vi "json Insert.vi"(8 "error in (no error)":errorcluster, 9 "anything":variant, 10 "path":string, 11 "JSON Document in":refnum<class "JSON Document.lvclass">) -> (0 "error out":errorcluster, 1 "replaced?":bool, 3 "JSON Document out":refnum<class "JSON Document.lvclass">)   [LabVIEW 2015, in "JSON Document.lvclass"]
uses:
  JSON Document.lvclass
  poly instances/json Insert I32 - string path.vi
  poly instances/json Insert I64 - string path.vi
  poly instances/json Insert U32 - string path.vi
  poly instances/json Insert U64 - string path.vi
  poly instances/json Insert Float - string path.vi
  poly instances/json Insert Double - string path.vi
  poly instances/json Insert Boolean - string path.vi
  poly instances/json Insert String - string path.vi
  poly instances/json Insert Path - string path.vi
  poly instances/json Insert json - string path.vi
  <vilib>/Utility/Data Type/NI_Data Type.lvlib
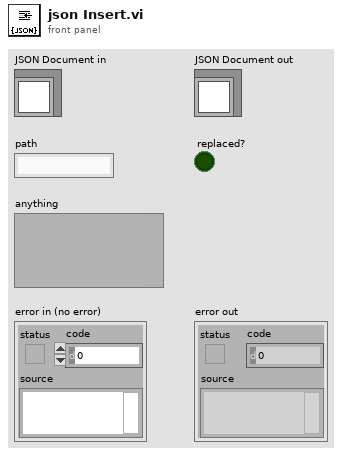
[diagram p1: front panel]
types:
  T1 = typedef "NI_Data Type.lvlib/Data Type.ctl" = enum8{"Invalid Type", "Void", "I8", "I16", "I32", "I64", "U8", "U16", "U32", "U64", "Single Float", "Double Float", "Extended Float", "Single Complex", "Double Complex", "Extended Complex", "Enum U8", "Enum U16", "Enum U32", "Enum U64", "Single Float With Unit", "Double Float With Unit", "Extended Float With Unit", "Single Complex with Unit", "Double Complex with Unit", "Extended Complex with Unit", "Boolean", "String", "Path", "Picture", "Tag", "Array", "Cluster", "Variant", "LV Variant", "Waveform", "Timestamp", "Digital Waveform", "Digital Data", "ExpressData", "Refnum", "External Data", "VI", "Poly VI", "LabVIEW Class Instance", "Fixed Point"}
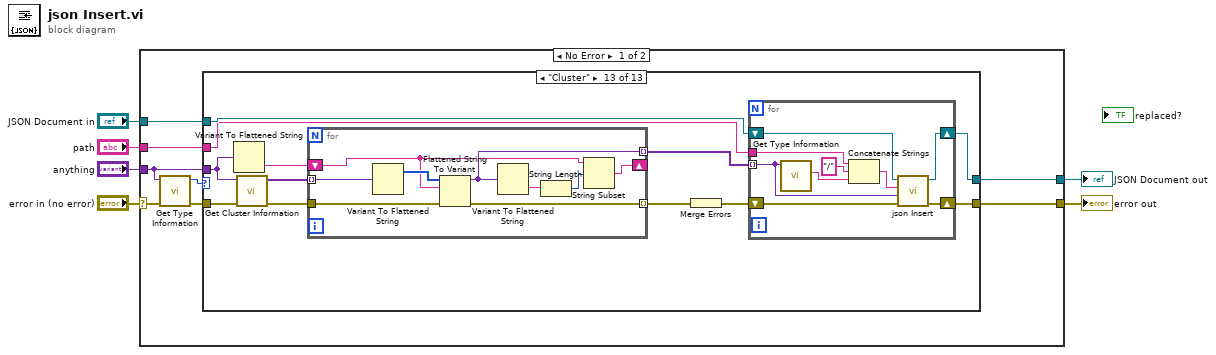
[diagram p0: block diagram]
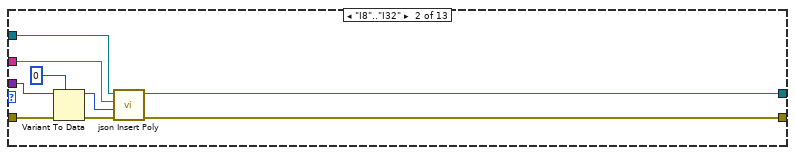
[diagram p3: hidden frame]
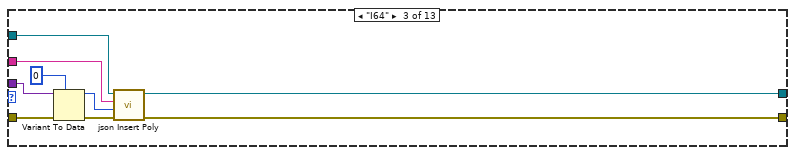
[diagram p4: hidden frame]
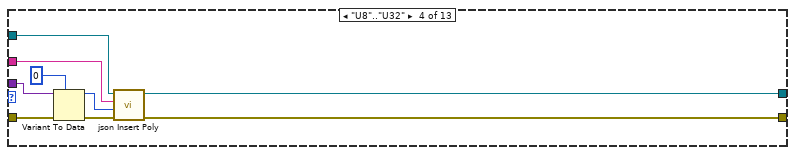
[diagram p5: hidden frame]
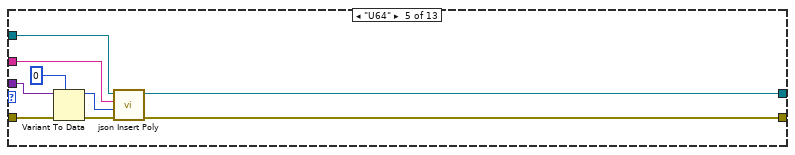
[diagram p6: hidden frame]
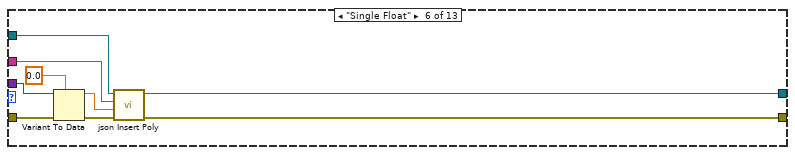
[diagram p7: hidden frame]
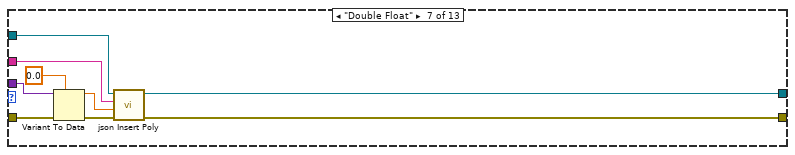
[diagram p8: hidden frame]
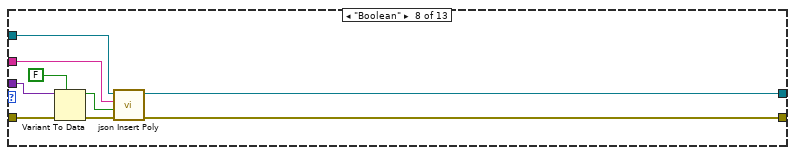
[diagram p9: hidden frame]
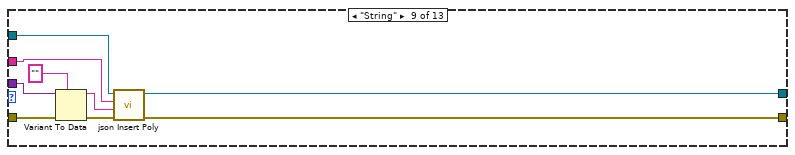
[diagram p10: hidden frame]
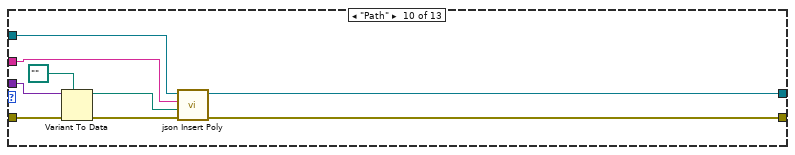
[diagram p11: hidden frame]
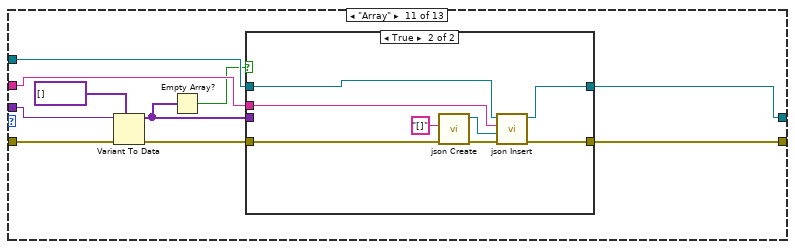
[diagram p12: hidden frame]
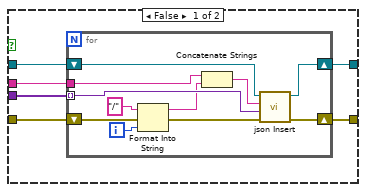
[diagram p13: hidden frame]
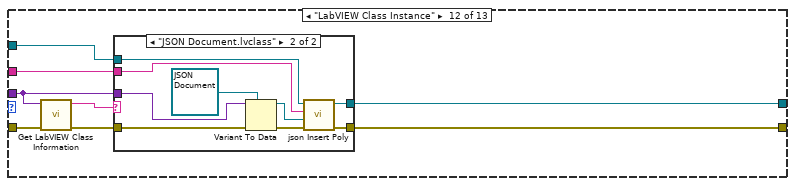
[diagram p14: hidden frame]
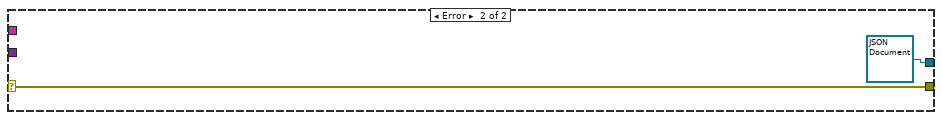
[diagram p16: hidden frame]
diagram:
  n1 = case shown="No Error" "error in (no error)" {
    selector: "error in (no error)" -> [w10 w182]
    tunnel: "anything" -> [w13 _]
    tunnel: [w11 refnum<class "JSON Document.lvclass"> refnum ("JSON Document out")] -> w4
    tunnel: [w9 w182] -> w3
    tunnel: "JSON Document in" -> [w8 _]
    tunnel: "path" -> [w7 _]
    frame No Error {
      n2 = call <vilib>:"Get Type Information.vi"("error in (no error)"=w10, "Variant"=w13) -> ("error out"=w12:errorcluster, "Type"=w14:T1)  [unwired: 5 in, 3 out]
      n3 = case shown="\"Cluster\"" w14 {
        tunnel: w13 -> [_ w24 w33 w42 w51 w60 w69 w78 w87 w96 w106 w138 w159]
        tunnel: w12 -> [w16 w23 w32 w41 w50 w59 w68 w77 w86 w95 w105 w140 w153]
        tunnel: w8 -> [w15 w21 w30 w39 w48 w57 w66 w75 w84 w93 w103 w136 w156]
        tunnel: [w15 w19 w28 w37 w46 w55 w64 w73 w82 w91 w102 w133 w155] -> w11
        tunnel: [w16 w18 w27 w36 w45 w54 w63 w72 w81 w90 w101 w134 w152] -> w9
        tunnel: w7 -> [_ w17 w26 w35 w44 w53 w62 w71 w80 w89 w100 w135 w154]
        frame "Invalid Type", Default {
        }
        frame "I8".."I32" {
          n4 = Variant To Data(error in=w23, type=0, Variant=w24) -> (data=w20:i32, error out=w22:errorcluster)
          n5 = call-poly "json Insert Poly.vi"("error in (no error)"=w22, "anything"=w20, "path"=w17, "JSON Document in"=w21) -> ("error out"=w18:errorcluster, "JSON Document out"=w19:refnum<class "JSON Document.lvclass">)  [unwired: 5 in, 1 out]
        }
        frame "I64" {
          n6 = Variant To Data(error in=w32, type=i64 0, Variant=w33) -> (data=w29:i64, error out=w31:errorcluster)
          n7 = call-poly "json Insert Poly.vi"("error in (no error)"=w31, "anything"=w29, "path"=w26, "JSON Document in"=w30) -> ("error out"=w27:errorcluster, "JSON Document out"=w28:refnum<class "JSON Document.lvclass">)  [unwired: 5 in, 1 out]
        }
        frame "U8".."U32" {
          n8 = Variant To Data(error in=w41, type=u32 0, Variant=w42) -> (data=w38:u32, error out=w40:errorcluster)
          n9 = call-poly "json Insert Poly.vi"("error in (no error)"=w40, "anything"=w38, "path"=w35, "JSON Document in"=w39) -> ("error out"=w36:errorcluster, "JSON Document out"=w37:refnum<class "JSON Document.lvclass">)  [unwired: 5 in, 1 out]
        }
        frame "U64" {
          n10 = Variant To Data(error in=w50, type=u64 0, Variant=w51) -> (data=w47:u64, error out=w49:errorcluster)
          n11 = call-poly "json Insert Poly.vi"("error in (no error)"=w49, "anything"=w47, "path"=w44, "JSON Document in"=w48) -> ("error out"=w45:errorcluster, "JSON Document out"=w46:refnum<class "JSON Document.lvclass">)  [unwired: 5 in, 1 out]
        }
        frame "Single Float" {
          n12 = Variant To Data(error in=w59, type=sgl 0.0, Variant=w60) -> (data=w56:sgl, error out=w58:errorcluster)
          n13 = call-poly "json Insert Poly.vi"("error in (no error)"=w58, "anything"=w56, "path"=w53, "JSON Document in"=w57) -> ("error out"=w54:errorcluster, "JSON Document out"=w55:refnum<class "JSON Document.lvclass">)  [unwired: 5 in, 1 out]
        }
        frame "Double Float" {
          n14 = Variant To Data(error in=w68, type=0.0, Variant=w69) -> (data=w65:dbl, error out=w67:errorcluster)
          n15 = call-poly "json Insert Poly.vi"("error in (no error)"=w67, "anything"=w65, "path"=w62, "JSON Document in"=w66) -> ("error out"=w63:errorcluster, "JSON Document out"=w64:refnum<class "JSON Document.lvclass">)  [unwired: 5 in, 1 out]
        }
        frame "Boolean" {
          n16 = Variant To Data(error in=w77, type=FALSE, Variant=w78) -> (data=w74:bool, error out=w76:errorcluster)
          n17 = call-poly "json Insert Poly.vi"("error in (no error)"=w76, "anything"=w74, "path"=w71, "JSON Document in"=w75) -> ("error out"=w72:errorcluster, "JSON Document out"=w73:refnum<class "JSON Document.lvclass">)  [unwired: 5 in, 1 out]
        }
        frame "String" {
          n18 = Variant To Data(error in=w86, type="", Variant=w87) -> (data=w83:string, error out=w85:errorcluster)
          n19 = call-poly "json Insert Poly.vi"("error in (no error)"=w85, "anything"=w83, "path"=w80, "JSON Document in"=w84) -> ("error out"=w81:errorcluster, "JSON Document out"=w82:refnum<class "JSON Document.lvclass">)  [unwired: 5 in, 1 out]
        }
        frame "Path" {
          n20 = Variant To Data(error in=w95, type=path "", Variant=w96) -> (data=w92:path, error out=w94:errorcluster)
          n21 = call-poly "json Insert Poly.vi"("error in (no error)"=w94, "anything"=w92, "path"=w89, "JSON Document in"=w93) -> ("error out"=w90:errorcluster, "JSON Document out"=w91:refnum<class "JSON Document.lvclass">)  [unwired: 5 in, 1 out]
        }
        frame "Array" {
          n22 = Variant To Data(error in=w105, type=variant[] [], Variant=w106) -> (data=w98:variant[], error out=w104:errorcluster)
          n23 = Empty Array?(array=w98) -> (empty?=w99:bool)
          n24 = case shown="True" w99 {
            tunnel: w104 -> [w113 w132]
            tunnel: w103 -> [w112 w131]
            tunnel: w98 -> [w111 _]
            tunnel: [w110 w130] -> w102
            tunnel: [w109 w129] -> w101
            tunnel: w100 -> [w108 w128]
            frame False {
              n25 = for {
                tunnel: w111 -> [w121] mode=indexing
                shift-right: [w123] -> w109
                shift-left: w113 -> [w115]
                shift-right: [w124] -> w110
                shift-left: w112 -> [w122]
                tunnel: w108 -> [w118]
                i -> [w120]
                n26 = Format Into String(initial string="/", error in=w115, w120) -> (resulting string=w117:string, error out=w114:errorcluster)  [unwired: 1 in]
                n27 = Concatenate Strings(w118, w117) -> (w116:string)
                n28 = call "json Insert.vi"("error in (no error)"=w114, "anything"=w121, "path"=w116, "JSON Document in"=w122) -> ("error out"=w123:errorcluster, "JSON Document out"=w124:refnum<class "JSON Document.lvclass">)  [unwired: 5 in, 1 out]
              }
            }
            frame True {
              n29 = call "json Create.vi"("error in (no error)"=w132, "JSON String"="[]") -> ("error out"=w126:errorcluster, "JSON Document out"=w127:refnum<class "JSON Document.lvclass">)  [unwired: 8 in]
              n30 = call "json Insert.vi"("error in (no error)"=w126, "anything"=w127, "path"=w128, "JSON Document in"=w131) -> ("error out"=w129:errorcluster, "JSON Document out"=w130:refnum<class "JSON Document.lvclass">)  [unwired: 5 in, 1 out]
            }
          }
        }
        frame "LabVIEW Class Instance" {
          n31 = call <vilib>:"Get LabVIEW Class Information.vi"("error in (no error)"=w140, "Variant"=w138) -> ("error out"=w137:errorcluster, "LabVIEW Class File Name"=w139:string)  [unwired: 7 in, 1 out]
          n32 = case shown="\"JSON Document.lvclass\"" w139 {
            tunnel: w138 -> [_ w151]
            tunnel: w137 -> [w141 w149]
            tunnel: w136 -> [w142 w148]
            tunnel: w135 -> [_ w147]
            tunnel: [w141 w144] -> w134
            tunnel: [w142 w143] -> w133
            frame "False", Default {
            }
            frame "JSON Document.lvclass" {
              n33 = Variant To Data(error in=w149, type=refnum<class "JSON Document.lvclass"> refnum ("JSON Document in"), Variant=w151) -> (data=w146:refnum<class "JSON Document.lvclass">, error out=w145:errorcluster)
              n34 = call-poly "json Insert Poly.vi"("error in (no error)"=w145, "anything"=w146, "path"=w147, "JSON Document in"=w148) -> ("error out"=w144:errorcluster, "JSON Document out"=w143:refnum<class "JSON Document.lvclass">)  [unwired: 5 in, 1 out]
            }
          }
        }
        frame "Cluster" {
          n35 = Variant To Flattened String(Variant=w159) -> (data string=w163:string)  [unwired: 1 out]
          n36 = call <vilib>:"Get Cluster Information.vi"("error in (no error)"=w153, "Variant"=w159) -> ("error out"=w161:errorcluster, "Cluster Elements"=w162:variant[])  [unwired: 8 in]
          n37 = for {
            tunnel: w162 -> [w181] mode=indexing
            tunnel: [w179] -> w158 mode=indexing
            shift-right: [w175] -> _
            shift-left: w163 -> [w178]
            tunnel: w161 -> [w174]
            tunnel: [w173] -> w160 mode=indexing
            n38 = Variant To Flattened String(Variant=w181) -> (1:w180:i16[])  [unwired: 1 out]
            n39 = Flattened String To Variant(4:w174, 6:w178, 7:w180) -> (0:w173:errorcluster, 3:w179:variant)
            n40 = Variant To Flattened String(Variant=w179) -> (data string=w177:string)  [unwired: 1 out]
            n41 = String Length(string=w177) -> (length=w176:i32)
            n42 = String Subset(string=w178, offset (0)=w176) -> (substring=w175:string)  [unwired: 1 in]
          }
          n43 = Merge Errors(w160) -> (w157:errorcluster)
          n44 = for {
            tunnel: w158 -> [w166] mode=indexing
            shift-right: [w171] -> w155
            shift-left: w156 -> [w172]
            tunnel: w154 -> [w170]
            shift-right: [w164] -> w152
            shift-left: w157 -> [w165]
            n45 = call <vilib>:"Get Type Information.vi"("Variant"=w166) -> ("Name"=w168:string)  [unwired: 6 in, 4 out]
            n46 = Concatenate Strings(w170, "/" ("string"), w168) -> (w167:string)
            n47 = call "json Insert.vi"("error in (no error)"=w165, "anything"=w166, "path"=w167, "JSON Document in"=w172) -> ("error out"=w164:errorcluster, "JSON Document out"=w171:refnum<class "JSON Document.lvclass">)  [unwired: 5 in, 1 out]
          }
        }
      }
    }
    frame Error {
    }
  }
  "error out" <- w3
  "JSON Document out" <- w4
